vi "Initialize.vi"(8 "error in (no error)":errorcluster, 11 "Class 1 in":refnum<class "csv.lvclass">) -> (0 "error out":errorcluster, 3 "Class 1 out":refnum<class "csv.lvclass">)   [LabVIEW 2021, in "Library.lvlib" / "csv.lvclass"]
uses:
  csv.lvclass
  csv.lvclass/csv.ctl
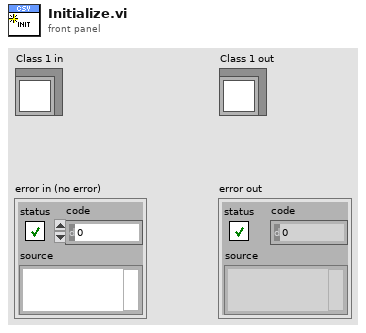
[diagram p1: front panel]
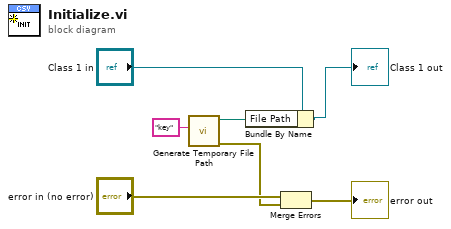
[diagram p0: block diagram]
diagram:
  n1 = call <vilib>:"Generate Temporary File Path.vi"("Temporary File Extension (tmp)"="key") -> ("error out"=w1:errorcluster, "Unique Temporary File Path"=w4:path)  [unwired: 9 in]
  n2 = Bundle By Name(cluster="Class 1 in", "File Path"=w4) -> (→"Class 1 out":refnum<class "csv.lvclass">)
  n3 = Merge Errors("error in (no error)", w1) -> (→"error out":errorcluster)
